vi "TelemetryServer_Initialize.vi"(9 "error in (no error)":errorcluster) -> (6 "error out":errorcluster, 7 "TelemetryServerPacket event":refnum<user-event>)   [LabVIEW 2009]
uses:
  TelemetryServer_Global.vi
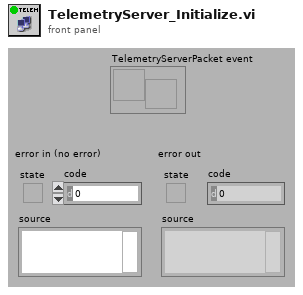
[diagram p1: front panel]
types:
  T1 = cluster{"Header":cluster{"lId":u32, "lSequenceNumber":u32, "lTimeFirstLow":u32, "lTimeFirstHigh":u32, "lTimeLastLow":u32, "lTimeLastHigh":u32, "dRate":dbl}, "mArrayDblHdl":dbl[], "mArrayExtHdl":ext[], "mArrayI16Hdl":i16[], "mArrayI32Hdl":i32[]}
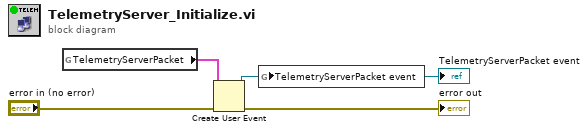
[diagram p0: block diagram]
diagram:
  n1 = global read "TelemetryServer_Global.vi" "TelemetryServerPacket"() -> (w2:T1)
  n2 = Create User Event(user event datatype=w2, error in="error in (no error)") -> (user event=w1:refnum<user-event>, error out=→"error out":errorcluster)
  "TelemetryServerPacket event" <- w1
  n3 = global write "TelemetryServer_Global.vi" "TelemetryServerPacket event"(w1) -> ()
